vi "BatterySettings2.vi"(4 "Battery Type":T1(ring)) -> (0 "RatedCapacity (Ah)":dbl=4.0, 1 "Min Voltage (V)":dbl=2.5, 2 "Max Voltage (V)":dbl=4.2)   [LabVIEW 2020]
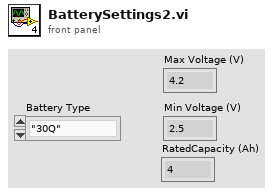
[diagram p1: front panel]
types:
  T1 = enum16{"\"30Q\"", "\"40T\"", "\"2P30Q\"", "\"3P30Q\"", "\"Nissan Leaf\""}
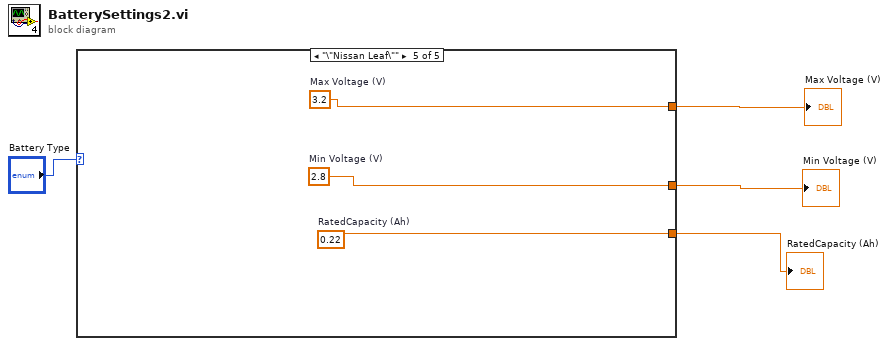
[diagram p0: block diagram]
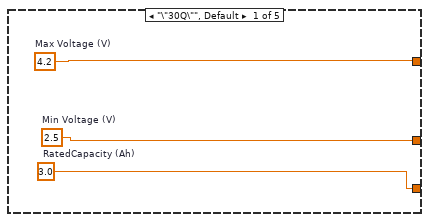
[diagram p2: hidden frame]
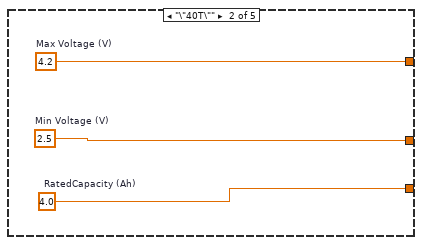
[diagram p3: hidden frame]
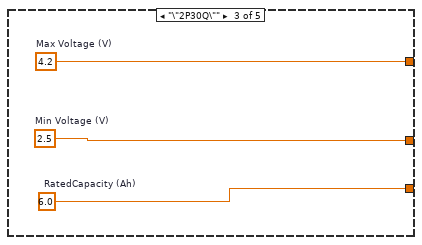
[diagram p4: hidden frame]
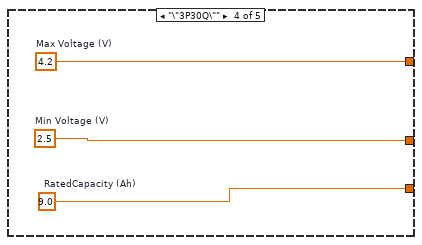
[diagram p5: hidden frame]
diagram:
  n1 = case shown="\"\\\"Nissan Leaf\\\"\"" "Battery Type" {
    tunnel: [w7 w10 w13 w16 w19] -> w4
    tunnel: [w6 w9 w12 w15 w17] -> w3
    tunnel: [w5 w8 w11 w14 w18] -> w2
    frame "\"30Q\"", Default {
      w5 = 3.0  # RatedCapacity (Ah)
      w6 = 4.2  # Max Voltage (V)
      w7 = 2.5  # Min Voltage (V)
    }
    frame "\"40T\"" {
      w8 = 4.0  # RatedCapacity (Ah)
      w9 = 4.2  # Max Voltage (V)
      w10 = 2.5  # Min Voltage (V)
    }
    frame "\"2P30Q\"" {
      w11 = 6.0  # RatedCapacity (Ah)
      w12 = 4.2  # Max Voltage (V)
      w13 = 2.5  # Min Voltage (V)
    }
    frame "\"3P30Q\"" {
      w14 = 9.0  # RatedCapacity (Ah)
      w15 = 4.2  # Max Voltage (V)
      w16 = 2.5  # Min Voltage (V)
    }
    frame "\"Nissan Leaf\"" {
      w18 = 0.22  # RatedCapacity (Ah)
      w17 = 3.2  # Max Voltage (V)
      w19 = 2.8  # Min Voltage (V)
    }
  }
  "Min Voltage (V)" <- w4
  "Max Voltage (V)" <- w3
  "RatedCapacity (Ah)" <- w2
